vi "test_shared_variable.vi"() -> ()   [LabVIEW 2017]
panel:
  in  "stop":bool
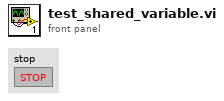
[diagram p1: front panel]
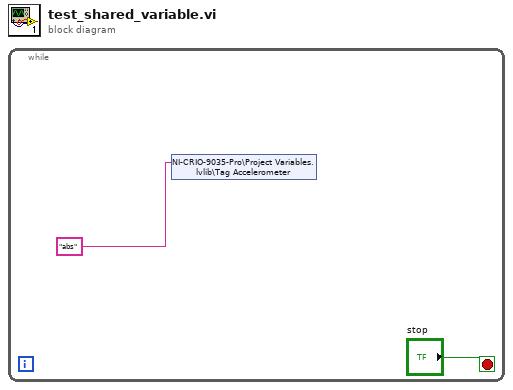
[diagram p0: block diagram]
diagram:
  n1 = while {
    stop <- "stop" stop-if-true
    n2 = shared-variable "NI-CRIO-9035-Pro\\Project Variables.lvlib\\Tag Accelerometer"("abs") -> ()  [unwired: 1 in, 1 out]
  }
